vi "Set_speed_and_move__2nd_XY_set_loacal_origin.vi"() -> ()   [LabVIEW 2015]
panel:
  out "Received String2 2":string="R\r\n"
  out "Received String1":string="OK\r\n"
  out "OK Done":bool=TRUE
  out "Received String2":string="R\r\n"
  out "String Received 2":string="OK\r\n"
  out "Command String 2":string="A:1+P400"
  out "OK move 1":bool=TRUE
  in  "Pulse Number 1":u32=100 min=1 max=500000
  in  "Axis Number 1":u8=1
  out "OK speed 1":bool=TRUE
  in  "Port Number":i8=3 min=0
  out "String Received":string="OK\r\n"
  out "Command String":string="D:1S1000F2000R100"
  in  "Acceleration Time":u16=100 max=1000
  in  "High Speed":u32=2000 min=1 max=500000
  in  "Low Speed":u32=1000 min=1 max=500000
  # "Set speed"
  # "Move to the absolute position"
  # "Abs. position Z\nin um"
  # "Z"
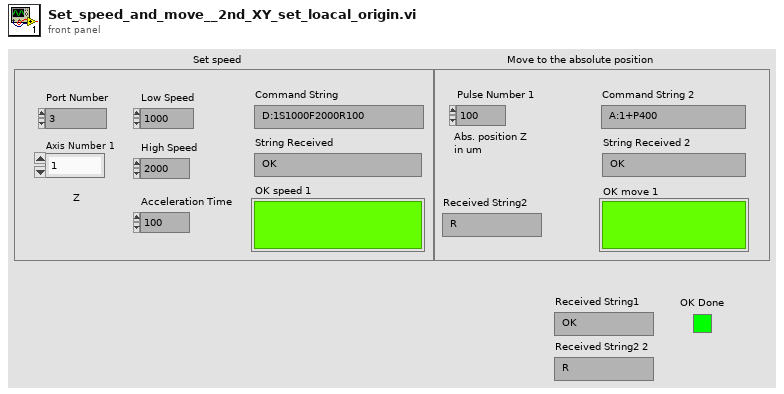
[diagram p1: front panel]
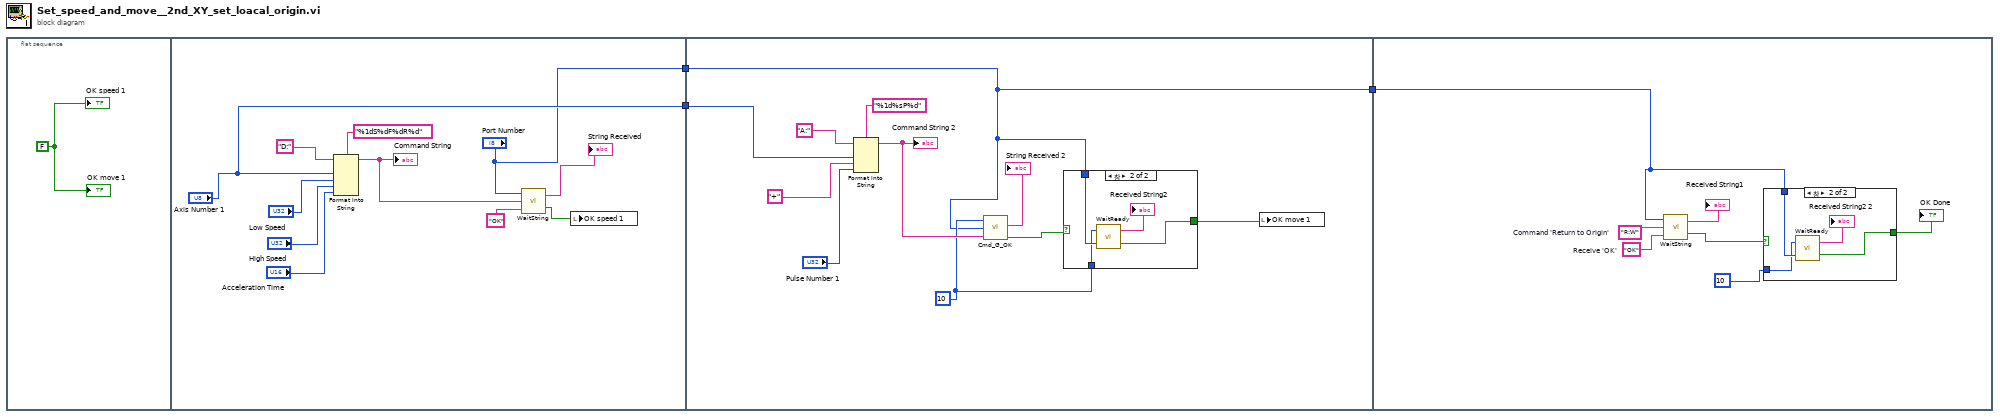
[diagram p0: block diagram]
diagram:
  n1 = flat-sequence {
    tunnel: ["Axis Number 1"] -> w3
    tunnel: ["Port Number"] -> w2
    tunnel: w3 -> [w19]
    tunnel: w2 -> [w16]
    tunnel: [w16] -> w1
    tunnel: w1 -> [w32]
    frame #0 {
      w4 = FALSE
      "OK speed 1" <- w4
      "OK move 1" <- w4
    }
    frame #1 {
      n2 = Format Into String(format string="%1dS%dF%dR%d", initial string="D:", "Axis Number 1", "Low Speed", "High Speed", "Acceleration Time") -> (resulting string=w9:string)  [unwired: 1 in, 1 out]
      "Command String" <- w9
      n3 = call "WaitString.vi"("String to Receive"="OK", "String to Send"=w9, "PortNumber"="Port Number") -> ("OK Done"=w5:bool, "String Received"=→"String Received":string)
      n4 = local write "OK speed 1"(w5) -> ()
    }
    frame #2 {
      w17 = 10
      n5 = Format Into String(format string="%1d%sP%d", initial string="A:", w19, "+", "Pulse Number 1") -> (resulting string=w23:string)  [unwired: 1 in, 1 out]
      "Command String 2" <- w23
      n6 = call "Cmd_G_OK.vi"("Residence time"=w17, "PortNumber"=w16, "Command String"=w23) -> ("Received String2"=→"String Received 2":string, "OK Done"=w25:bool)  [unwired: 2 out]
      n7 = case shown="참" w25 {
        selector: w25 -> [w27 _]
        tunnel: w16 -> [_ w31]
        tunnel: [w27 w29] -> w18
        tunnel: w17 -> [_ w28]
        frame False {
        }
        frame True {
          n8 = call "WaitReady.vi"("PortNumber"=w31, "Residence time in ms"=w28) -> ("OK Done"=w29:bool, "String Received"=→"Received String2":string)
        }
      }
      n9 = local write "OK move 1"(w18) -> ()
    }
    frame #3 {
      w33 = "OK"  # Receive 'OK'
      w34 = "R:W"  # Command 'Return to Origin'
      n10 = call "WaitString.vi"("String to Receive"=w33, "String to Send"=w34, "PortNumber"=w32) -> ("OK Done"=w36:bool, "String Received"=→"Received String1":string)
      n11 = case shown="참" w36 {
        selector: w36 -> [w39 _]
        tunnel: w32 -> [_ w43]
        tunnel: [w39 w41] -> w38
        tunnel: 10 -> [_ w40]
        frame False {
        }
        frame True {
          n12 = call "WaitReady.vi"("PortNumber"=w43, "Residence time in ms"=w40) -> ("OK Done"=w41:bool, "String Received"=→"Received String2 2":string)
        }
      }
      "OK Done" <- w38
    }
  }
